vi "LCC Set Sw Scaling On.vi"(7 "Scaling On":bool, 8 "error in (no error)":errorcluster caption="Fehler (Eingang, kein Fehler)", 11 "Channel Handle":i64) -> (0 "error out":errorcluster caption="Fehler (Ausgang)")   [LabVIEW 2021, in "labbCAN_Controller_API.lvlib"]
doc: "LCC_Func long LCC_CALL LCC_SetSwScalingOn(dev_hdl ChanHdl,\n unsigned char ScalingOn);"
uses:
  labbCAN_Controller_API.lvlib
  labbCAN_Controller_API.dll
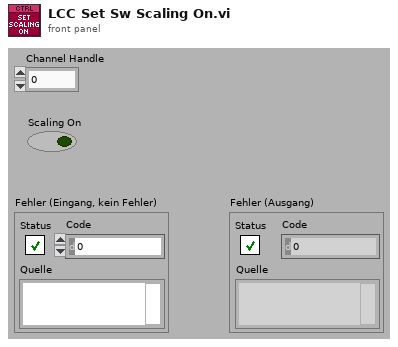
[diagram p1: front panel]
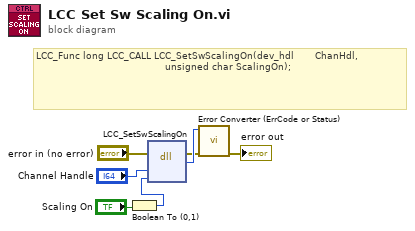
[diagram p0: block diagram]
diagram:
  # "LCC_Func long LCC_CALL LCC_SetSwScalingOn(dev_hdl       ChanHdl,\n                                           unsigned char ScalingOn);"
  n1 = Boolean To (0,1)(Boolean="Scaling On") -> (0, 1=w1:i16)
  n2 = dll-call lib="C:/Users/olaja/AppData/Local/CETONI_SDK/labbCAN_Controller_API.*" fn="LCC_SetSwScalingOn"(error in="error in (no error)", "ChanHdl"="Channel Handle", "ScalingOn"=w1) -> (error out=w4:errorcluster, "Rückgabetyp"=w5:i32)  [unwired: 4 in, 1 out]
  n3 = call "Error Converter (ErrCode or Status).vi"("error in (no error)"=w4, "error code"=w5) -> ("error out"=→"error out":errorcluster)  [unwired: 9 in]
